vi "test Parse Sorted Object Dictionary_2.vi"(11 "Test Case In":refnum<class "test EDS.lvclass">) -> (0 "error out":errorcluster, 3 "Test Case Out":refnum<class "test EDS.lvclass">)   [LabVIEW 2024, in "test EDS.lvclass"]
uses:
  test EDS.lvclass
  C:/Program Files/National Instruments/LabVIEW 2024/vi.lib/Astemes/LUnit/Test Case.lvclass
  Core/EDS/EDS.lvclass
  Core/Object Type.ctl
  Core/Data Type.ctl
  Core/Access Type.ctl
  Core/EDS/EDS.lvclass/EDS.ctl
  <vilib>/Astemes/LUnit/Test Case.lvclass/Test Case.ctl
  <vilib>/Astemes/LUnit/Append Fail Result.vi
  <vilib>/Astemes/LUnit/Append Pass Result.vi
  <vilib>/Astemes/LUnit/Run In UI.vi
  <vilib>/Utility/error.llb/Clear Errors.vi
  Core/OD Sub-Entry/OD Sub-Entry.lvclass
  D:/git/EDS-File-Viewer/Core/OD Entry/OD Entry.lvclass
  Core/Sorted Object Dictionary/Sorted Object Dictionary.lvclass
  Core/OD Entry/OD Entry.lvclass
  <vilib>/Astemes/LUnit/Test Case.lvclass
  Core/EDS.lvlib
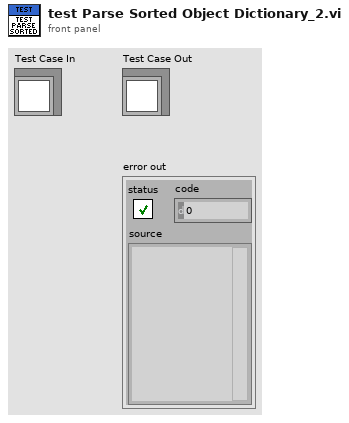
[diagram p1: front panel]
types:
  T1 = typedef "EDS.lvlib/Access Type.ctl" = enum16{"ro", "wo", "rw", "rwr", "rww", "const"}
  T2 = typedef "EDS.lvlib/Data Type.ctl" = u16
  T3 = typedef "EDS.lvlib/Object Type.ctl" = u8
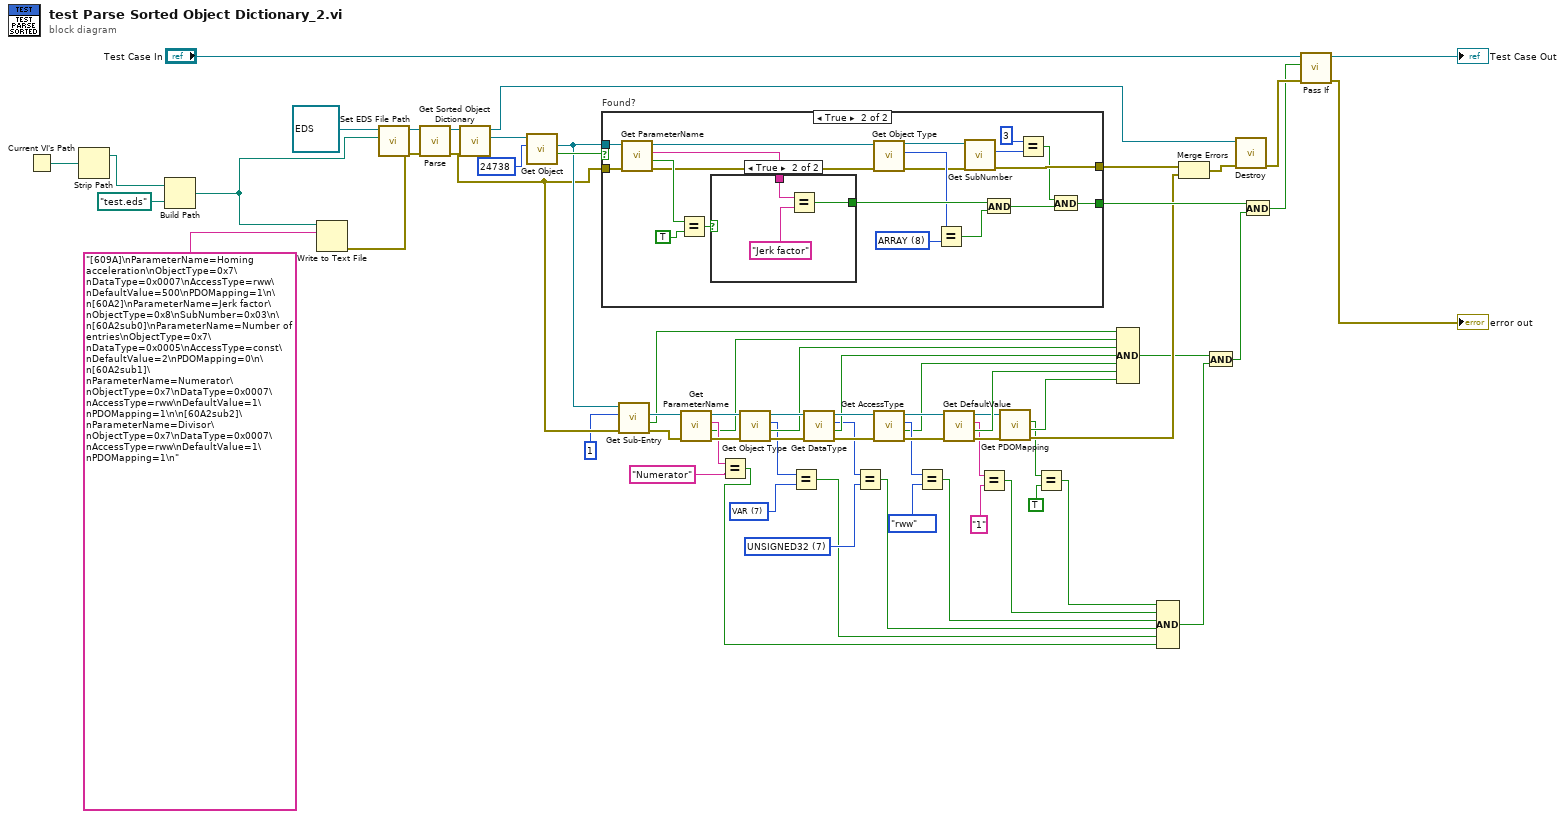
[diagram p0: block diagram]
diagram:
  w24 = T2 7 items=["BOOLEAN"=1, "INTEGER8"=2, "INTEGER16"=3, "INTEGER32"=4, "UNSIGNED8"=5, "UNSIGNED16"=6, "UNSIGNED32"=7, "REAL32"=8, "VISIBLE_STRING"=9, "OCTET_STRING"=10, "UNICODE_STRING"=11, "TIME_OF_DAY"=12, "TIME_DIFFERENCE"=13, "RESERVED1"=14, "DOMAIN"=15, "INTEGER24"=16, "REAL64"=17, "INTEGER40"=18, "INTEGER48"=19, "INTEGER56"=20, "INTEGER64"=21, "UNSIGNED24"=22, "RESERVED2"=23, "UNSIGNED40"=24, "UNSIGNED48"=25, "UNSIGNED56"=26, "UNSIGNED64"=27, "RESERVED3"=28, "RESERVED4"=29, "RESERVED5"=30, "RESERVED6"=31, "PDO_COMMUNICATION_PARAMETER"=32, "PDO_MAPPING"=33, "SDO_PARAMETER"=34, "IDENTITY"=35, "RESERVED7"=36] ("DataType")
  w26 = T3 7 items=["NULL"=0, "DOMAIN"=2, "DEFTYPE"=5, "DEFSTRUCT"=6, "VAR"=7, "ARRAY"=8, "RECORD"=9] ("ObjectType")
  n1 = Current VI's Path() -> (path=w60:path)
  n2 = Strip Path(path=w60) -> (stripped path=w56:path)  [unwired: 1 out]
  n3 = Build Path(base path=w56, name or relative path=path "test.eds") -> (appended path=w57:path)
  n4 = Write to Text File(file (use dialog)=w57, text="[609A]\nParameterName=Homing acceleration\nObjectType=0x7\nDataType=0x0007\nAccessType=rww\nDefaultValue=500\nPDOMapping=1\n\n[60A2]\nParameterName=Jerk factor\nObjectType=0x8\nSubNumber=0x03\n\n[60A2sub0]\nParameterName=Number of entries\nObjectType=0x7\nDataType=0x0005\nAccessType=const\nDefaultValue=2\nPDOMapping=0\n\n[60A2sub1]\nParameterName=Numerator\nObjectType=0x7\nDataType=0x0007\nAccessType=rww\nDefaultValue=1\nPDOMapping=1\n\n[60A2sub2]\nParameterName=Divisor\nObjectType=0x7\nDataType=0x0007\nAccessType=rww\nDefaultValue=1\nPDOMapping=1\n") -> (error out=w58:errorcluster)  [unwired: 2 in, 2 out]
  n5 = call "Set EDS File Path.vi"("EDS File Path"=w57, "EDS in"=refnum<class "EDS.lvclass"> refnum ("EDS.lvlib:EDS.lvclass")) -> ("EDS out"=w61:refnum<class "EDS.lvclass">)  [unwired: 9 in]
  n6 = call "Parse.vi"("error in"=w58, "EDS in"=w61) -> ("error out"=w45:errorcluster, "EDS out"=w55:refnum<class "EDS.lvclass">)  [unwired: 8 in]
  n7 = call "Get Sorted Object Dictionary.vi"("EDS in"=w55) -> ("Sorted Object Dictionary"=w52:refnum<class "Sorted Object Dictionary.lvclass">, "EDS out"=w54:refnum<class "EDS.lvclass">)  [unwired: 9 in]
  n8 = call "Get Object.vi"("Numeric"=u16 24738, "Sorted Object Dictionary in"=w52) -> ("Found?"=w47:bool, "OD Entry"=w46:refnum<class "OD Entry.lvclass">)  [unwired: 7 in, 1 out]
  n9 = case "Found?" shown="True" w47 {
    selector: w47 -> [w66 _]
    tunnel: w46 -> [_ w87]
    tunnel: w45 -> [w67 w86]
    tunnel: [w66 w69] -> w50
    tunnel: [w67 w73] -> w48
    frame False {
    }
    frame True {
      w77 = T3 8 items=["NULL"=0, "DOMAIN"=2, "DEFTYPE"=5, "DEFSTRUCT"=6, "VAR"=7, "ARRAY"=8, "RECORD"=9] ("y")
      n10 = call "Get ParameterName.vi"("Error In"=w86, "reference in"=w87) -> ("Error Out"=w79:errorcluster, "Defined?"=w85:bool, "ParameterName"=w83:string, "reference out"=w80:refnum<class "OD Entry.lvclass">)  [unwired: 6 in]
      n11 = Equal?(x=w85, y=TRUE) -> (x = y?=w82:bool)
      n12 = case shown="True" w82 {
        selector: w82 -> [w88 _]
        tunnel: w83 -> [_ w91]
        tunnel: [w88 w89] -> w81
        frame False {
        }
        frame True {
          n13 = Equal?(x=w91, y="Jerk factor") -> (x = y?=w89:bool)
        }
      }
      n14 = call "Get Object Type.vi"("Error In"=w79, "reference in"=w80) -> ("Error Out"=w74:errorcluster, "ObjectType"=w78:T3, "reference out"=w72:refnum<class "OD Entry.lvclass">)  [unwired: 6 in, 1 out]
      n15 = Equal?(x=w78, y=w77) -> (x = y?=w75:bool)
      n16 = call "Get SubNumber.vi"("Error In"=w74, "reference in"=w72) -> ("Error Out"=w73:errorcluster, "SubNumber"=w71:u8)  [unwired: 6 in, 2 out]
      n17 = And(x=w81, y=w75) -> (x .and. y?=w76:bool)
      n18 = Equal?(x=u8 3, y=w71) -> (x = y?=w68:bool)
      n19 = And(x=w68, y=w76) -> (x .and. y?=w69:bool)
    }
  }
  n20 = call "Get Sub-Entry.vi"("Error In"=w45, "Sub-Index"=u16 1, "reference in"=w46) -> ("Error Out"=w43:errorcluster, "Found?"=w31:bool, "OD Sub-Entry"=w44:refnum<class "OD Sub-Entry.lvclass">)  [unwired: 5 in, 1 out]
  n21 = call "Get ParameterName.vi"("Error In"=w43, "reference in"=w44) -> ("Error Out"=w42:errorcluster, "Defined?"=w30:bool, "ParameterName"=w33:string, "reference out"=w41:refnum<class "OD Sub-Entry.lvclass">)  [unwired: 6 in]
  n22 = Equal?(x=w33, y="Numerator") -> (x = y?=w6:bool)
  n23 = call "Get Object Type.vi"("Error In"=w42, "reference in"=w41) -> ("Error Out"=w39:errorcluster, "Defined?"=w29:bool, "ObjectType"=w27:T3, "reference out"=w40:refnum<class "OD Sub-Entry.lvclass">)  [unwired: 6 in]
  n24 = Equal?(x=w27, y=w26) -> (x = y?=w5:bool)
  n25 = call "Get DataType.vi"("Error In"=w39, "reference in"=w40) -> ("Error Out"=w36:errorcluster, "Set?"=w28:bool, "DataType"=w25:T2, "reference out"=w37:refnum<class "OD Sub-Entry.lvclass">)  [unwired: 6 in]
  n26 = Equal?(x=w25, y=w24) -> (x = y?=w4:bool)
  n27 = call "Get AccessType.vi"("Error In"=w36, "reference in"=w37) -> ("Error Out"=w34:errorcluster, "Defined?"=w21:bool, "AccessType"=w23:T1, "reference out"=w35:refnum<class "OD Sub-Entry.lvclass">)  [unwired: 6 in]
  n28 = Equal?(x=w23, y=Access_Type."rww") -> (x = y?=w3:bool)
  n29 = call "Get DefaultValue.vi"("Error In"=w34, "reference in"=w35) -> ("Error Out"=w17:errorcluster, "Set?"=w20:bool, "DefaultValue"=w15:string, "reference out"=w18:refnum<class "OD Sub-Entry.lvclass">)  [unwired: 6 in]
  n30 = Equal?(x=w15, y="1") -> (x = y?=w2:bool)
  n31 = call "Get PDOMapping.vi"("Error In"=w17, "reference in"=w18) -> ("Error Out"=w16:errorcluster, "Defined?"=w19:bool, "PDOMapping"=w13:bool)  [unwired: 6 in, 1 out]
  n32 = Equal?(x=w13, y=TRUE) -> (x = y?=w1:bool)
  n33 = Compound Arithmetic op=AND(w31, w30, w29, w28, w21, w20, w19) -> (w9:bool)
  n34 = Compound Arithmetic op=AND(w1, w2, w3, w4, w5, w6) -> (w7:bool)
  n35 = Merge Errors(w48, w16) -> (w11:errorcluster)
  n36 = And(x=w9, y=w7) -> (x .and. y?=w8:bool)
  n37 = call "Destroy.vi"("error in"=w11, "EDS in"=w54) -> ("error out"=w49:errorcluster)  [unwired: 8 in, 1 out]
  n38 = And(x=w50, y=w8) -> (x .and. y?=w10:bool)
  n39 = call <vilib>:"Pass If.vi"("error in (no error)"=w49, "Pass?"=w10, "LUnit Test Case In"="Test Case In") -> ("error out"=→"error out":errorcluster, "LUnit Test Case Out"=→"Test Case Out":refnum<class "test EDS.lvclass">)  [unwired: 7 in]
